vi "Test Join Split.vi"() -> ()   [LabVIEW 2021]
uses:
  DataTypes_CIF_U.lvlib
panel:
  out "Pass":bool
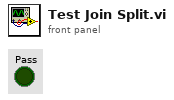
[diagram p1: front panel]
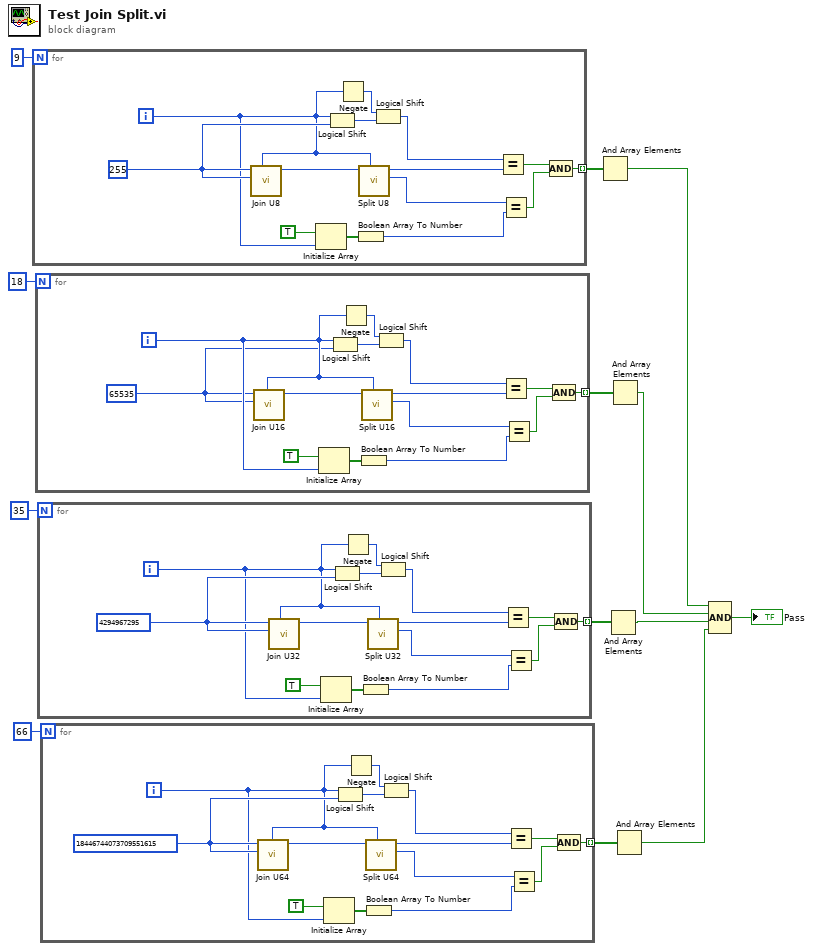
[diagram p0: block diagram]
diagram:
  n1 = for {
    N: 9 -> [_]
    tunnel: [w22] -> w6 mode=indexing
    i -> [w16]
    w17 = u8 255 ("MSB")
    n2 = call "Join U8.vi"("LSB Length"=w16, "LSB"=w17, "MSB"=w17) -> ("U8"=w18:u8)  [unwired: 8 in]
    n3 = Initialize Array(TRUE, w16) -> (w20:bool[])
    n4 = Logical Shift(y=w16, x=w17) -> (x << y=w27:u8)
    n5 = Negate(x=w16) -> (-x=w25:i32)
    n6 = Boolean Array To Number(Boolean array=w20) -> (number=w19:u64)
    n7 = call "Split U8.vi"("LSB Length"=w16, "U8"=w18) -> ("LSB"=w14:u8, "MSB"=w15:u8)  [unwired: 8 in]
    n8 = Logical Shift(y=w25, x=w27) -> (x << y=w26:u8)
    n9 = Equal?(x=w26, y=w15) -> (x = y?=w23:bool)
    n10 = Equal?(x=w14, y=w19) -> (x = y?=w24:bool)
    n11 = Compound Arithmetic op=AND(w23, w24) -> (w22:bool)
  }
  n12 = for {
    N: 18 -> [_]
    tunnel: [w36] -> w7 mode=indexing
    i -> [w29]
    w28 = u16 65535 ("MSB")
    n13 = call "Join U16.vi"("LSB Length"=w29, "LSB"=w28, "MSB"=w28) -> ("U16"=w32:u16)  [unwired: 8 in]
    n14 = Initialize Array(TRUE, w29) -> (w34:bool[])
    n15 = Logical Shift(y=w29, x=w28) -> (x << y=w41:u16)
    n16 = Negate(x=w29) -> (-x=w39:i32)
    n17 = Boolean Array To Number(Boolean array=w34) -> (number=w33:u16)
    n18 = call "Split U16.vi"("LSB Length"=w29, "U16"=w32) -> ("LSB"=w31:u16, "MSB"=w30:u16)  [unwired: 8 in]
    n19 = Logical Shift(y=w39, x=w41) -> (x << y=w40:u16)
    n20 = Equal?(x=w40, y=w30) -> (x = y?=w37:bool)
    n21 = Equal?(x=w31, y=w33) -> (x = y?=w38:bool)
    n22 = Compound Arithmetic op=AND(w37, w38) -> (w36:bool)
  }
  n23 = for {
    N: 35 -> [_]
    tunnel: [w50] -> w8 mode=indexing
    i -> [w42]
    w45 = u32 4294967295 ("MSB")
    n24 = call "Join U32.vi"("LSB Length"=w42, "LSB"=w45, "MSB"=w45) -> ("U32"=w46:u32)  [unwired: 8 in]
    n25 = Initialize Array(TRUE, w42) -> (w48:bool[])
    n26 = Logical Shift(y=w42, x=w45) -> (x << y=w55:u32)
    n27 = Negate(x=w42) -> (-x=w53:i32)
    n28 = Boolean Array To Number(Boolean array=w48) -> (number=w47:u32)
    n29 = call "Split U32.vi"("LSB Length"=w42, "U32"=w46) -> ("LSB"=w43:u32, "MSB"=w44:u32)  [unwired: 8 in]
    n30 = Logical Shift(y=w53, x=w55) -> (x << y=w54:u32)
    n31 = Equal?(x=w54, y=w44) -> (x = y?=w51:bool)
    n32 = Equal?(x=w43, y=w47) -> (x = y?=w52:bool)
    n33 = Compound Arithmetic op=AND(w51, w52) -> (w50:bool)
  }
  n34 = for {
    N: 66 -> [_]
    tunnel: [w62] -> w12 mode=indexing
    i -> [w56]
    w67 = u64 18446744073709551615 ("MSB")
    n35 = call "Join U64.vi"("LSB Length"=w56, "LSB"=w67, "MSB"=w67) -> ("U64"=w69:u64)  [unwired: 8 in]
    n36 = Initialize Array(TRUE, w56) -> (w58:bool[])
    n37 = Logical Shift(y=w56, x=w67) -> (x << y=w68:u64)
    n38 = Negate(x=w56) -> (-x=w65:i32)
    n39 = Boolean Array To Number(Boolean array=w58) -> (number=w57:u64)
    n40 = call "Split U64.vi"("LSB Length"=w56, "U64"=w69) -> ("LSB"=w60:u64, "MSB"=w61:u64)  [unwired: 8 in]
    n41 = Logical Shift(y=w65, x=w68) -> (x << y=w66:u64)
    n42 = Equal?(x=w66, y=w61) -> (x = y?=w63:bool)
    n43 = Equal?(x=w60, y=w57) -> (x = y?=w64:bool)
    n44 = Compound Arithmetic op=AND(w63, w64) -> (w62:bool)
  }
  n45 = And Array Elements(Boolean array=w6) -> (logical AND=w1:bool)
  n46 = And Array Elements(Boolean array=w8) -> (logical AND=w3:bool)
  n47 = And Array Elements(Boolean array=w7) -> (logical AND=w2:bool)
  n48 = And Array Elements(Boolean array=w12) -> (logical AND=w4:bool)
  n49 = Compound Arithmetic op=AND(w1, w2, w3, w4) -> (→"Pass":bool)
